vi "AmpToRing.vi"(11 "Amplitude":sgl) -> (3 "Ring Value":u8)   [LabVIEW 2012, in "StimulCtrls.lvlib"]
uses:
  StimulCtrls.lvlib
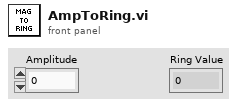
[diagram p1: front panel]
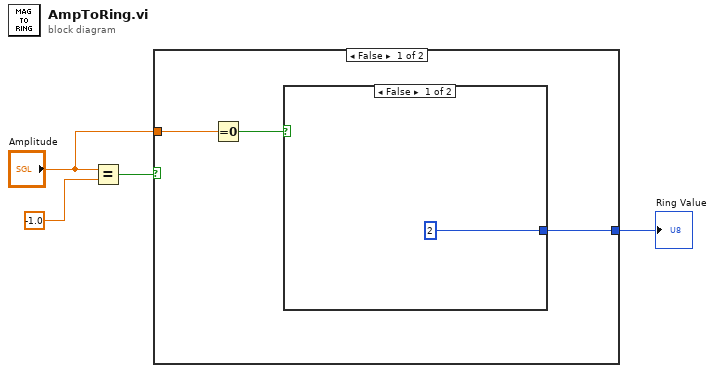
[diagram p0: block diagram]
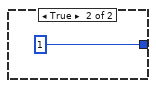
[diagram p2: hidden frame]
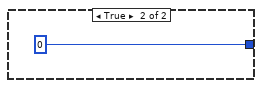
[diagram p3: hidden frame]
diagram:
  n1 = Equal?(x="Amplitude", y=sgl -1.0) -> (x = y?=w3:bool)
  n2 = case shown="False" w3 {
    tunnel: [w5 0] -> w2
    tunnel: "Amplitude" -> [w7 _]
    frame False {
      n3 = Equal To 0?(x=w7) -> (x = 0?=w6:bool)
      n4 = case shown="False" w6 {
        tunnel: [2 1] -> w5
        frame False {
        }
        frame True {
        }
      }
    }
    frame True {
    }
  }
  "Ring Value" <- w2
